vi "Draw Omni Wheel.vi"(6 "wheel state":T1, 7 "picture info":T3={"picture size"={"Width"=500, "Height"=500}, "pixels per unit"=10.0}, 8 "error in (no error)":errorcluster, 9 "draw wheel options":T2={"global wheel position"={"x"=0.0, "y"=0.0}, "wheel frame angle (rad)"=0.0, "color (black)"=0, "draw wheel state"=FALSE, "draw forward velocity"=FALSE, "velocity scale"=16711680.0, "velocity color (red)"=16711680}, 10 "picture in":picture, 11 "wheel in":refnum<class "NI_Robotics_Wheel.lvclass">) -> (0 "error out":errorcluster, 2 "picture out":picture, 3 "wheel out":refnum<class "NI_Robotics_Wheel.lvclass">)   [LabVIEW 2017, in "NI_Robotics_Steering Picture.lvlib"]
uses:
  <vilib>/robotics/Utilities/Visualization/Steering Visualization/Steering Picture/NI_Robotics_Steering Picture.lvlib
  <vilib>/robotics/Steering/Wheel/NI_Robotics_Wheel.lvclass
  <vilib>/robotics/Utilities/Visualization/Steering Visualization/Steering Picture/Picture Info.ctl
  <vilib>/Utility/miscctls.llb/LVBoundsTypeDef.ctl
  <vilib>/robotics/Utilities/Visualization/Steering Visualization/Steering Picture/Draw Wheel Options.ctl
  <vilib>/robotics/Steering/Wheel/Wheel State.ctl
  <vilib>/Analysis/coordinate.llb/2D Cartesian Coordinate Rotation.vi
  <vilib>/Analysis/coordinate.llb/2D Cartesian Coordinate Rotation (Array).vi
  <vilib>/robotics/Utilities/Visualization/Steering Visualization/Steering Picture/Global Position to Pixel.vi
  <vilib>/Analysis/coordinate.llb/Angle Rotation.vi
  <vilib>/Analysis/coordinate.llb/Angle Rotation (scalar).vi
  <vilib>/Analysis/coordinate.llb/Wrap Angle (scalar).vi
  <vilib>/picture/picture.llb/Draw Line.vi
  <vilib>/picture/picture.llb/Move Pen.vi
  <vilib>/picture/picture.llb/Draw Point.vi
  <vilib>/picture/picture.llb/Draw Multiple Lines.vi
  <vilib>/robotics/Steering/Wheel/Get Omnidirectional Wheel Information.vi
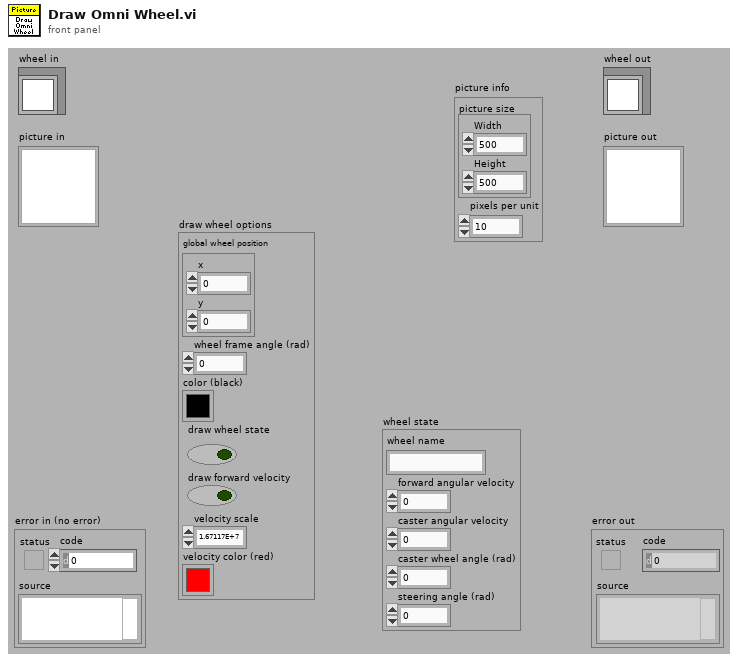
[diagram p1: front panel]
types:
  T1 = typedef "NI_Robotics_Wheel.lvclass/Wheel State.ctl" = cluster{"wheel name":string, "forward angular velocity":dbl, "caster angular velocity":dbl, "caster wheel angle (rad)":dbl, "steering angle (rad)":dbl}
  T2 = typedef "NI_Robotics_Steering Picture.lvlib/Draw Wheel Options.ctl" = cluster{"global wheel position":cluster{"x":dbl, "y":dbl}, "wheel frame angle (rad)":dbl, "color (black)":u32, "draw wheel state":bool, "draw forward velocity":bool, "velocity scale":dbl, "velocity color (red)":u32}
  T3 = typedef "NI_Robotics_Steering Picture.lvlib/Picture Info.ctl" = cluster{"picture size":T4, "pixels per unit":dbl}
  T4 = typedef "LVBoundsTypeDef.ctl" = cluster{"Width":u32, "Height":u32}
  T5 = typedef "NI_Robotics_Wheel.lvclass/Wheel Parameters.ctl" = cluster{"wheel radius":dbl, "gear ratio":dbl, "forward rotation direction":T6}
  T6 = typedef "NI_Robotics_Wheel.lvclass/Rotation Direction.ctl" = u16
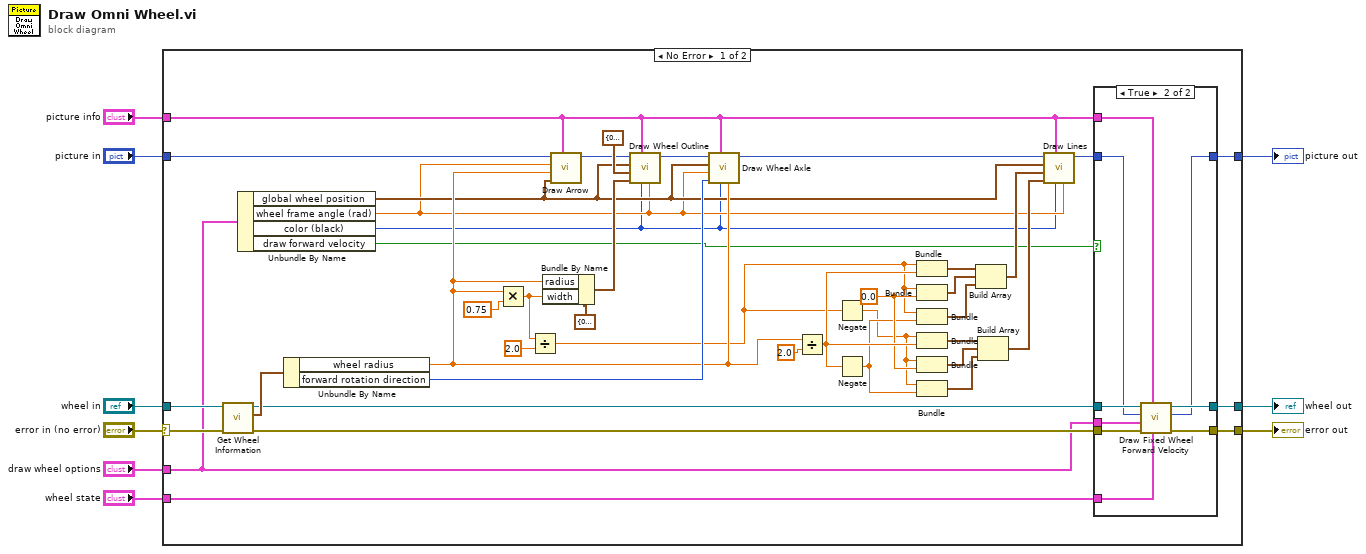
[diagram p0: block diagram]
diagram:
  n1 = case shown="No Error" "error in (no error)" {
    selector: "error in (no error)" -> [w50 w66]
    tunnel: [w16 w66] -> w8
    tunnel: "wheel in" -> [w51 w64]
    tunnel: "picture info" -> [w13 _]
    tunnel: "picture in" -> [w41 w65]
    tunnel: [w14 w65] -> w5
    tunnel: [w18 w64] -> w4
    tunnel: "draw wheel options" -> [w10 _]
    tunnel: "wheel state" -> [w11 _]
    frame No Error {
      w34 = 0.0 ("y")
      n2 = call-poly <vilib>:"Get Wheel Information.vi"("error in (no error)"=w50, "wheel in"=w51) -> ("error out"=w17:errorcluster, "wheel parameters"=w42:T5, "wheel out"=w19:refnum<class "NI_Robotics_Wheel.lvclass">)  [unwired: 5 in, 2 out]
      n3 = Unbundle By Name(w10) -> ("global wheel position"=w22:cluster{"x":dbl, "y":dbl}, "wheel frame angle (rad)"=w21:dbl, "color (black)"=w20:u32, "draw forward velocity"=w12:bool)
      n4 = Unbundle By Name(w42) -> ("wheel radius"=w37:dbl, "forward rotation direction"=w43:T6)
      n5 = Multiply(x=w37, y=0.75) -> (x*y=w40:dbl)
      n6 = Divide(x=w40, y=2.0) -> (x/y=w32:dbl)
      n7 = Bundle By Name(cluster=cluster{"radius":dbl, "width":dbl} {"radius"=0.0, "width"=0.0} ("size"), "radius"=w37, "width"=w40) -> (w48:cluster{"radius":dbl, "width":dbl})
      n8 = call <vilib>:"Draw Arrow.vi"("picture info"=w13, "global base position"=w22, "length"=w37, "wheel frame angle (rad)"=w21, "picture in"=w41) -> ("picture out"=w44:picture)  [unwired: 6 in]
      n9 = call <vilib>:"Draw Wheel Outline.vi"("angle (rad)"=w21, "color (black)"=w20, "picture info"=w13, "size"=w48, "offset from center"=cluster{"x":dbl, "y":dbl} {"x"=0.0, "y"=0.0}, "global wheel position"=w22, "picture in"=w44) -> ("picture out"=w45:picture)  [unwired: 4 in]
      n10 = call <vilib>:"Draw Wheel Axle.vi"("length"=w37, "color (black)"=w20, "picture info"=w13, "rotation direction"=w43, "wheel frame angle (rad)"=w21, "global wheel position"=w22, "picture in"=w45) -> ("picture out"=w36:picture)  [unwired: 4 in]
      n11 = Divide(x=w37, y=2.0) -> (x/y=w35:dbl)
      n12 = Negate(x=w32) -> (-x=w31:dbl)
      n13 = Negate(x=w35) -> (-x=w33:dbl)
      n14 = Bundle(w32, w35) -> (w30:cluster{dbl, dbl})  [unwired: 1 in]
      n15 = Bundle(w32, "y"=w34) -> (w29:cluster{dbl, "y":dbl})  [unwired: 1 in]
      n16 = Bundle(w32, w33) -> (w28:cluster{dbl, dbl})  [unwired: 1 in]
      n17 = Bundle(w31, w35) -> (w27:cluster{dbl, dbl})  [unwired: 1 in]
      n18 = Bundle(w31, "y"=w34) -> (w26:cluster{dbl, "y":dbl})  [unwired: 1 in]
      n19 = Bundle(w31, w33) -> (w25:cluster{dbl, dbl})  [unwired: 1 in]
      n20 = Build Array(w30, w29, w28) -> (w24:cluster{dbl, "y":dbl}[])
      n21 = Build Array(w27, w26, w25) -> (w23:cluster{dbl, "y":dbl}[])
      n22 = call <vilib>:"Draw Lines.vi"("wheel frame angle (rad)"=w21, "color (black)"=w20, "picture info"=w13, "end points"=w23, "start points"=w24, "global wheel position"=w22, "picture in"=w36) -> ("picture out"=w15:picture)  [unwired: 4 in]
      n23 = case shown="True" w12 {
        tunnel: w19 -> [w53 w63]
        tunnel: [w53 w62] -> w18
        tunnel: w17 -> [w52 w61]
        tunnel: [w52 w60] -> w16
        tunnel: w15 -> [w54 w59]
        tunnel: [w54 w58] -> w14
        tunnel: w13 -> [_ w57]
        tunnel: w11 -> [_ w56]
        tunnel: w10 -> [_ w55]
        frame False {
        }
        frame True {
          n24 = call <vilib>:"Draw Fixed Wheel Forward Velocity.vi"("wheel state"=w56, "picture info"=w57, "error in (no error)"=w61, "draw wheel options"=w55, "picture in"=w59, "wheel in"=w63) -> ("error out"=w60:errorcluster, "picture out"=w58:picture, "wheel out"=w62:refnum<class "NI_Robotics_Wheel.lvclass">)  [unwired: 3 in]
        }
      }
    }
    frame Error {
    }
  }
  "error out" <- w8
  "wheel out" <- w4
  "picture out" <- w5
